vi "limits_checkCondition.vi"(7 "Sec":i32, 8 "error in (no error)":errorcluster, 9 "user event out":T1, 10 "Data in":T2[](array[typedef]), 11 "test limits":T3[](array[typedef])) -> (0 "error out":errorcluster, 2 "Data out":T2[](array[typedef]))   [LabVIEW 2019]
uses:
  limits_limitList.ctl
  limits_specs.ctl
  core/core_autoMonitorDataCluster.ctl
  gui/test_result_user_event.ctl
  report_mode.ctl
  <vilib>/Analysis/baseanly.llb/Mean (DBL).vi
  <vilib>/Analysis/NI_AALBase.lvlib
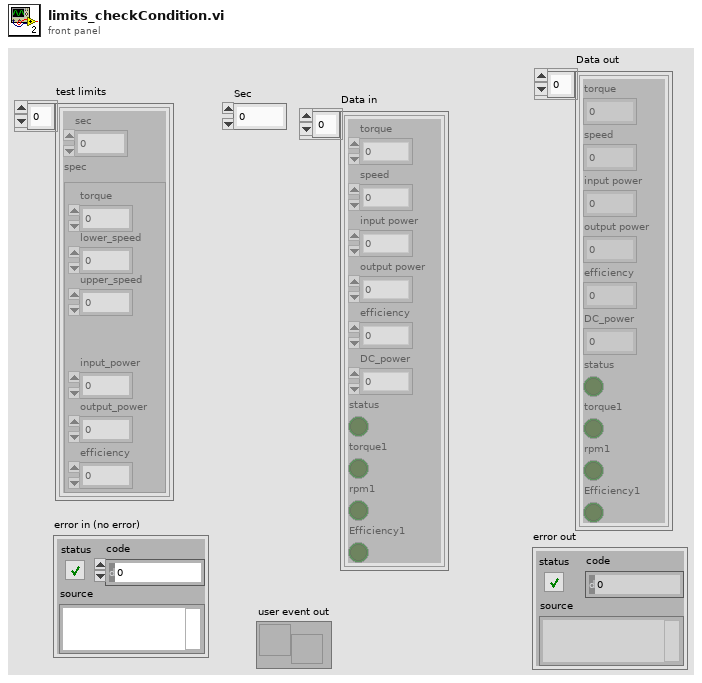
[diagram p1: front panel]
types:
  T1 = typedef "test_result_user_event.ctl" = refnum<user-event>
  T2 = typedef "core_autoMonitorDataCluster.ctl" = cluster{"torque":dbl, "speed":dbl, "input power":dbl, "output power":dbl, "efficiency":dbl, "DC_power":dbl, "status":bool, "torque1":bool, "rpm1":bool, "Efficiency1":bool}
  T3 = typedef "limits_limitList.ctl" = cluster{"sec":i32, "spec":T4}
  T4 = typedef "limits_specs.ctl" = cluster{"torque":dbl, "lower_speed":dbl, "upper_speed":dbl, "input_power":dbl, "output_power":dbl, "efficiency":dbl}
  T5 = typedef "report_mode.ctl" = enum16{"Initialize", "Save", "Close"}
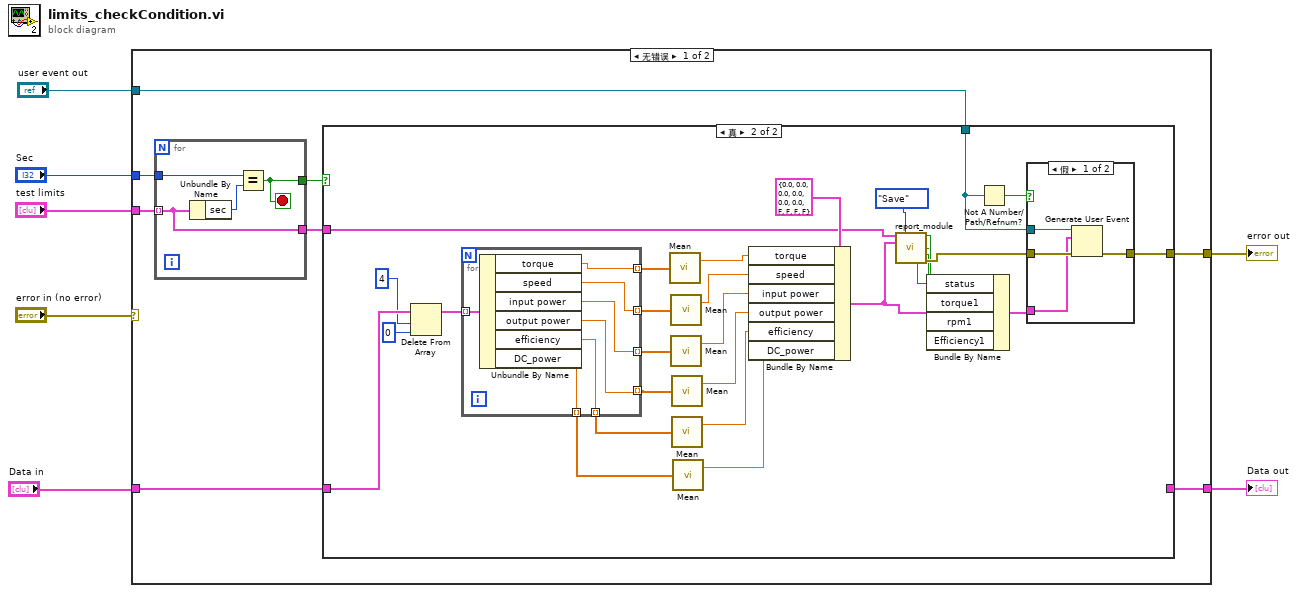
[diagram p0: block diagram]
diagram:
  n1 = case shown="无错误" "error in (no error)" {
    selector: "error in (no error)" -> [_ w62]
    tunnel: "test limits" -> [w15 _]
    tunnel: "Sec" -> [w14 _]
    tunnel: "Data in" -> [w12 _]
    tunnel: [w11 w62] -> w3
    tunnel: [w9 _] -> w2
    tunnel: "user event out" -> [w8 _]
    frame No Error {
      n2 = for {
        tunnel: w15 -> [w59] mode=indexing
        tunnel: w14 -> [w58]
        tunnel: [w60] -> w13
        tunnel: [w59] -> w10
        stop <- w60 stop-if-true
        n3 = Unbundle By Name(w59) -> ("sec"=w61:i32)
        n4 = Equal?(x=w58, y=w61) -> (x = y?=w60:bool)
      }
      n5 = case shown="真" w13 {
        tunnel: w12 -> [w16 w29]
        tunnel: [_ w33] -> w11
        tunnel: w10 -> [_ w21]
        tunnel: [w16 _] -> w9
        tunnel: w8 -> [_ w32]
        frame False {
        }
        frame True {
          n6 = Delete From Array(array=w29, length=4 ("长度"), index=0 ("索引")) -> (array with subset deleted=w28:T2[])  [unwired: 1 out]
          n7 = for {
            tunnel: w28 -> [w57] mode=indexing
            tunnel: [w56] -> w45 mode=indexing
            tunnel: [w55] -> w44 mode=indexing
            tunnel: [w54] -> w43 mode=indexing
            tunnel: [w53] -> w42 mode=indexing
            tunnel: [w52] -> w41 mode=indexing
            tunnel: [w51] -> w34 mode=indexing
            n8 = Unbundle By Name(w57) -> ("torque"=w56:dbl, "speed"=w55:dbl, "input power"=w54:dbl, "output power"=w53:dbl, "efficiency"=w52:dbl, "DC_power"=w51:dbl)
          }
          n9 = call-poly <vilib>:"Mean.vi"("X"=w45) -> ("mean"=w40:dbl)  [unwired: 1 out]
          n10 = call-poly <vilib>:"Mean.vi"("X"=w44) -> ("mean"=w39:dbl)  [unwired: 1 out]
          n11 = call-poly <vilib>:"Mean.vi"("X"=w43) -> ("mean"=w38:dbl)  [unwired: 1 out]
          n12 = call-poly <vilib>:"Mean.vi"("X"=w42) -> ("mean"=w37:dbl)  [unwired: 1 out]
          n13 = call-poly <vilib>:"Mean.vi"("X"=w41) -> ("mean"=w36:dbl)  [unwired: 1 out]
          n14 = call-poly <vilib>:"Mean.vi"("X"=w34) -> ("mean"=w35:dbl)  [unwired: 1 out]
          n15 = Bundle By Name(cluster=T2 {"torque"=0.0, "speed"=0.0, "input power"=0.0, "output power"=0.0, "efficiency"=0.0, "DC_power"=0.0, "status"=FALSE, "torque1"=FALSE, "rpm1"=FALSE, "Efficiency1"=FALSE} ("AutoMonitorCluster"), "torque"=w40, "speed"=w39, "input power"=w38, "output power"=w37, "efficiency"=w36, "DC_power"=w35) -> (w23:T2)
          n16 = call "report_module.vi"("limits"=w21, "mode"=report_mode."Save", "data"=w23) -> ("Torque"=w20:bool, "Rpm"=w19:bool, "Efficiency"=w18:bool, "step status"=w25:bool, "error out"=w24:errorcluster)  [unwired: 7 in, 1 out]
          n17 = Bundle By Name(cluster=w23, "status"=w25, "torque1"=w20, "rpm1"=w19, "Efficiency1"=w18) -> (w17:T2)
          n18 = Not A Number/Path/Refnum?(number/path/refnum=w32) -> (NaN/Path/Refnum?=w31:bool)
          n19 = case shown="假" w31 {
            tunnel: [w49 w50] -> w33
            tunnel: w32 -> [w48 _]
            tunnel: w24 -> [w47 w50]
            tunnel: w17 -> [w46 _]
            frame False {
              n20 = Generate User Event(user event=w48, event data cluster=w46, error in=w47) -> (error out=w49:errorcluster)  [unwired: 1 in, 1 out]
            }
            frame True {
            }
          }
        }
      }
    }
    frame Error {
    }
  }
  "error out" <- w3
  "Data out" <- w2
